vi "Dashboard Main.vi"() -> ()   [LabVIEW 2019]
uses:
  <vilib>/Utility/miscctls.llb/LVRowAndColumnTypeDef.ctl
  <vilib>/event_ctls.llb/eventvkey.ctl
  <vilib>/Rock Robotics/Network Tables/NT Read Numeric Array.vi
  <vilib>/Rock Robotics/Network Tables/NT Write Boolean.vi
  <vilib>/Rock Robotics/WPI/Dashboard/WPI_DashboardLogging Global.vi
panel:
  out "Background":bool
  in  "Camera Settings Right":T1={"Frame Rate"=30, "Compression"=30, "Size"=1, "DB Camera Config"=FALSE} {"Frame Rate" scale=1.0..30.0; "Compression" scale=100.0..-1.0; "Size" items=["640x480", "320x240", "160x120"]}
  in  "Camera Name Right":string(combo)="No Camera Selection"
  out "Camera Perf":string
  in  "Camera Settings":T1={"Frame Rate"=30, "Compression"=30, "Size"=1, "DB Camera Config"=FALSE} {"Frame Rate" scale=1.0..30.0; "Compression" scale=100.0..-1.0; "Size" items=["640x480", "320x240", "160x120"]}
  in  "TCP":refnum<k5>
  in  "Rec Mode":enum32{"Stop", "Record", "Playback"}(radio)
  out "Robot IP":string
  out "Image Message":string="Timeout in Camera Communications"
  in  "Dashboard Tab":T2(tab)
  in  "Select Auto":string(combo)="Select Autonomous ..."
  out "NT Connection":bool
  out "MotorChart R":cluster{"Numeric":dbl, "Numeric":dbl}(graph)
  out "MotorChart L":cluster{"Numeric":dbl, "Numeric":dbl}(graph)
  out "MotorSliders R":cluster{"MotorSlide1":dbl, "MotorSlide2":dbl} {"MotorSlide2" scale=-1.0..1.0 scale format="%#_2e"; "MotorSlide1" scale=-1.0..1.0 scale format="%#_2e"}
  out "MotorSliders L":cluster{"MotorSlide1":dbl, "MotorSlide2":dbl} {"MotorSlide2" scale=-1.0..1.0 scale format="%#_2e"; "MotorSlide1" scale=-1.0..1.0 scale format="%#_2e"}
  out "Gyro":dbl(knob) scale=0.0..360.0
  out "JS1 Z":dbl(slide) scale=-1.0..1.0 scale format="%#_2e"
  out "JS1 Graph":cluster{"X":dbl, "Y":dbl}[](graph)
  out "JS1 Buttons":T3
  out "JS2 Z":dbl(slide) scale=-1.0..1.0 scale format="%#_2e"
  out "JS2 Graph":cluster{"X":dbl, "Y":dbl}[](graph)
  out "JS2 Buttons":T3
  out "Mode":T4(ring)=enum."Auto Disabled"
  out "Right Camera Perf":cluster{"Bandwidth (Mbps)":dbl, "FPS":dbl}
  out "Camera Image Right":T5(plugin-control)
  in  "DB/String 9":string
  in  "DB/String 8":string
  in  "DB/String 7":string
  in  "DB/String 6":string
  in  "DB/String 5":string
  in  "DB/String 4":string
  in  "DB/String 3":string
  in  "DB/String 2":string
  in  "DB/String 1":string
  in  "DB/String 0":string
  in  "DB/Slider 0":dbl(slide) scale=0.0..5.0
  in  "DB/Slider 1":dbl(slide) scale=0.0..5.0
  in  "DB/Slider 2":dbl(slide) scale=0.0..5.0
  in  "DB/Slider 3":dbl(slide) scale=0.0..5.0
  out "DB/LED 3":bool
  out "DB/LED 2":bool
  out "DB/LED 1":bool
  out "DB/LED 0":bool
  in  "DB/Button 3":bool
  in  "DB/Button 2":bool
  in  "DB/Button 1":bool
  in  "DB/Button 0":bool caption="New Name"
  in  "OK Button":bool
  out "Danger Light":bool
  in  "Cowbell Mode":bool
  out "Hyperdrive":string
  out "Motor Mode":string
  out "Color":string
  out "Encoder 2":dbl(knob) scale=0.0..360.0
  out "Encoder 1":dbl(knob) scale=0.0..360.0
  in  "Relay":bool
  in  "Test Slider":dbl(slide) scale=0.0..100.0 scale format="%#_3g"
  in  "On/Off":bool caption="Solenoid"
  in  "Test Name":u16(ring) items=["Select the test to run..."]
  in  "Test Tree":string(tree)
  in  "Motor":cluster{"Value":dbl, "Enable":bool} {"Value" scale=-1.0..1.0 scale format="%#_3g"}
  out "Progress":T6 {"Test Progress" scale=0.0..100.0}
  in  "Rev/Fwd":cluster{"Forward":bool, "Reverse":bool}
  in  "Test Ring":u16(ring) items=["Monochrome", "Color"]
  out "Cmd Status":string
  in  "Execute Command":bool
  in  "Command Params":string[][](table)
  in  "Command Selection":i32(listbox)
  in  "CheckList":i32(listbox)
  out "Tree":string(tree)
  out "Camera Image":T5(plugin-control)
  in  "Camera Name":string(combo)="No Camera Selection"
  # "HW"
  # "HW"
  # "Joysticks"
  # "Drive Motors"
  # "Front"
  # "Right"
  # "Left"
  # "Back"
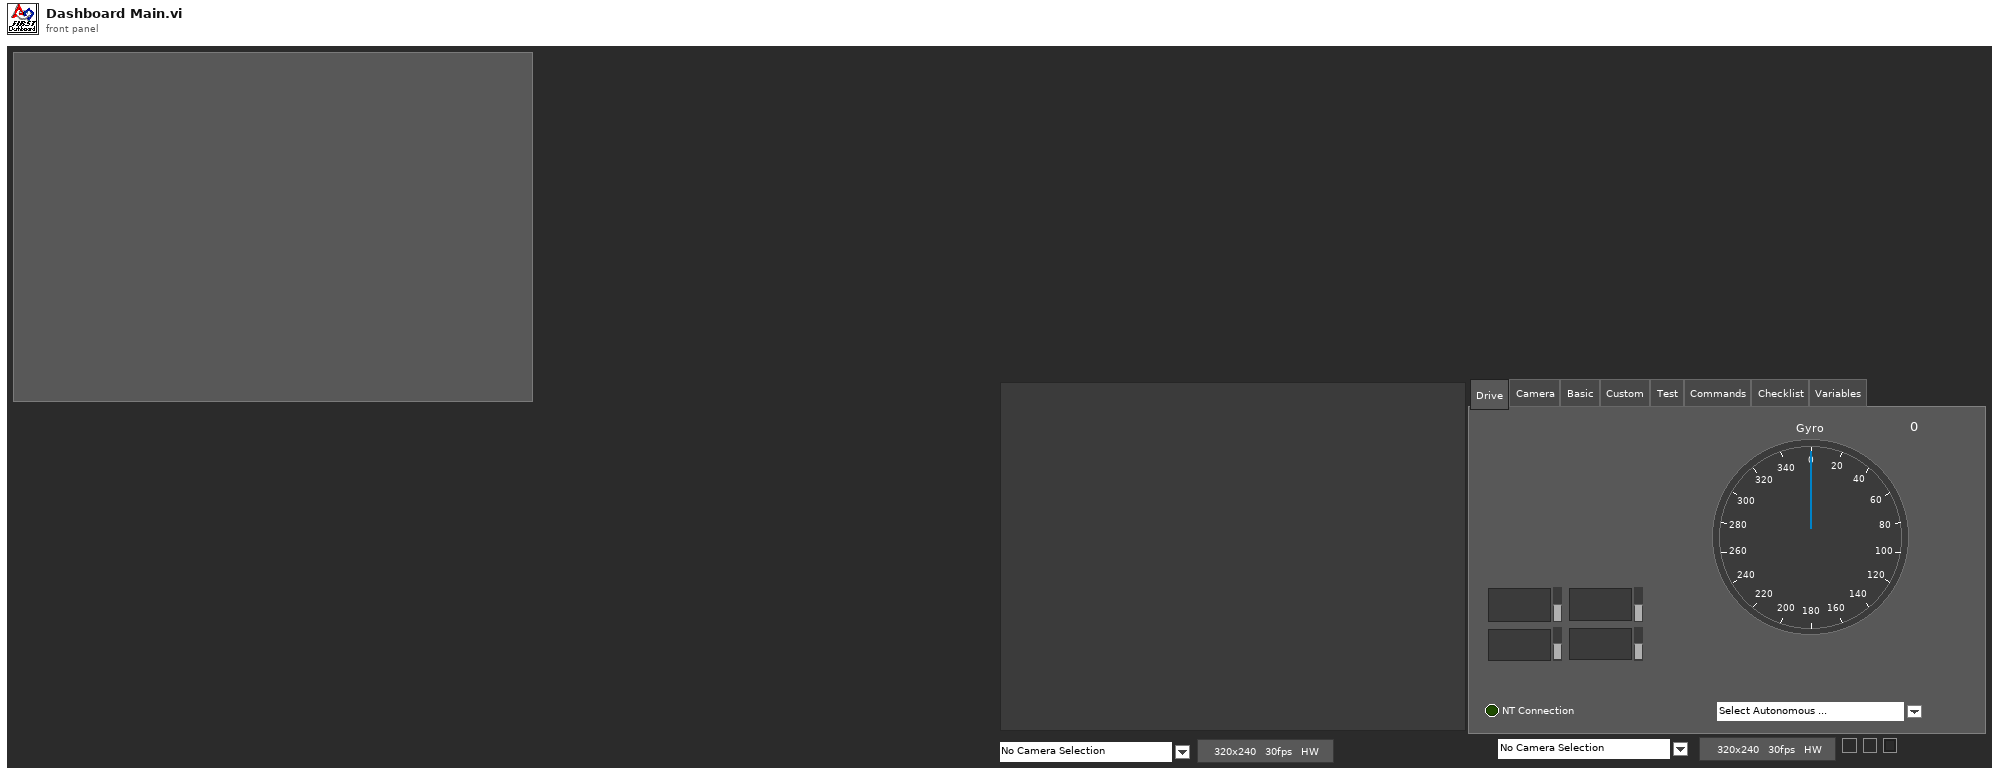
[diagram p1: front panel]
types:
  T1 = cluster{"Frame Rate":i32, "Compression":i32, "Size":u16, "DB Camera Config":bool}
  T2 = enum32{"Drive", "Camera", "Basic", "Custom", "Test", "Commands", "Checklist", "Variables"}
  T3 = cluster{bool, bool, bool, bool, bool, bool, bool, bool, bool, bool, bool, bool}
  T4 = enum8{"Tele-Op Disabled", "Tele-Op Enabled", "Auto Disabled", "Auto Enabled", "Test Disabled", "Test Enabled", "Disconnected", "No Code", "E-Stop"}
  T5 = typedef "IMAQ Image.ctl" = refnum<image>
  T6 = cluster{"Test Progress":u8, "Test Progress Text":string}
  T7 = cluster{"Save Path":path, "Interval (s)":dbl, "Keep":i32}
  T8 = typedef "Image Type" = u32
  T9 = cluster{"IDs":cluster{"RPC field ID":u16, "Unique ID":u16}, "String":string}
  T10 = cluster{"Global Rectangle":i32[], "Contours":cluster{"Contour Type":u32, "ROI Type":u32, "Points":i32[]}[]}
  T11 = cluster{"Camera Name":string, string, "Saved DB Images Info":cluster{"Save Path":path, "Interval (s)":dbl, "Keep":i32}}
  T12 = cluster{"Camera Name Right":string, string, "Saved DB Images Info":cluster{"Save Path":path, "Interval (s)":dbl, "Keep":i32}}
  T13 = cluster{"Camera Image":refnum<vi>, "Dashboard Tab":refnum<vi>, "Background":refnum<vi>, "Rec Mode":refnum<vi>, "Test Slider":refnum<vi>, "On/Off ":refnum<vi>, "Test Ring":refnum<vi>, "Rev/Fwd":refnum<vi>, "Test Name":refnum<vi>, "Motor":refnum<vi>, "Progress":refnum<vi>, "CheckList":refnum<vi>, "Tree":refnum<vi>, "Test Tree":refnum<vi>, "Command Params":refnum<vi>, "Command Selection":refnum<vi>, "Execute Command":refnum<vi>, "Cmd Status":refnum<vi>, "Camera Settings":refnum<vi>, "Camera Name":refnum<vi>, "Camera Perf":refnum<vi>, "Camera Settings Right":refnum<vi>, "Camera Name Right":refnum<vi>, "Camera Image Right":refnum<vi>}
  T14 = cluster{"Error Strings":string, "Disable Counts":cluster{u16, u16}, "Rail Faults":cluster{u16, u16, u16}, "Robot IP":string, "DB Mode":u8, "Event Info":cluster{"Name":string, "Type":u8, "Number":u16, "Replay":u8}}
  T15 = cluster{"Storage":cluster{"Disk Free":u64, "RAM Block":u32, "RAM free":u32}, "CPU Utilization":cluster{"CPU % ISR":sgl, "CPU % Time Crit":sgl, "CPU % Timed Str":sgl, "CPU % High":sgl, "CPU % Above":sgl, "CPU % Normal":sgl, "CPU % Low":sgl}, "CAN":cluster{"% Bus Utilization":sgl, "Bus Off Cnt":u32, "TX_FIFO Full Cnt":u32, "Receive Error Cnt":u8, "Transmit Error Cnt":u8}, "HID":cluster{"HID Outputs":u32, "Rumble Low":u16, "Rumble High":u16}[]}
  T16 = cluster{"Status bits":cluster{"Test Mode":bool, "Autonomous":bool, "Enabled":bool, "Code Start":bool, "Brownout":bool, "Reserved 2":bool, "Reserved 3":bool, "E-Stop":bool}, "Code Trace":cluster{"Disabled":bool, "TeleOp":bool, "Auto":bool, "Test":bool}, "Controller Type":enum16{"unknown", "cRIO", "roboRio"}, "Code?":enum16{"unknown", "noCode", "code"}, "Battery V":dbl}
  T17 = cluster{"Control Bits":cluster{"TestMode":bool, "Autonomous":bool, "Enabled":bool, "FMS Present":bool, bool, bool, bool, "E-Stop":bool}, "Team Station ":u8, "Countdown":sgl, "Joystick Values":cluster{"Axes":dbl[], "Buttons":bool[], "POVs":i16[]}[]}
  T18 = cluster{"Axes":dbl[], "Buttons":bool[], "POVs":i16[]}[]
  T19 = cluster{"Axes":dbl[], "Buttons":bool[], "POVs":i16[]}
  T20 = cluster{"Buttons[0]":bool, "Buttons[1]":bool, "Buttons[2]":bool, "Buttons[3]":bool, "Buttons[4]":bool, "Buttons[5]":bool, "Buttons[6]":bool, "Buttons[7]":bool, "Buttons[8]":bool, "Buttons[9]":bool, "Buttons[10]":bool, "Buttons[11]":bool}
  T21 = cluster{"Operation":enum16{"Update", "Clear"}, "Color Box":u32}[]
  T22 = typedef "eventvkey.ctl" = enum16{"ASCII", "Enter", "Return", "Shift", "Ctrl", "Alt", "Cmd", "Opt", "Caps", "NumLock", "Clear", "Break", "Up", "Down", "Left", "Right", "Insert", "Delete", "Home", "End", "PageUp", "PageDown", "Escape", "Help", "Pause", "ScrollLock", "F1", "F2", "F3", "F4", "F5", "F6", "F7", "F8", "F9", "F10", "F11", "F12", "F13", "F14", "F15", "F16", "F17", "F18", "F19", "F20", "F21", "F22", "F23", "F24", "Play", "VolumeUp", "VolumeDown", "Mute", "Two Byte Char"}
  T23 = cluster{"Image Size":bool, "Image Type":bool, "Pixel Value":bool, "ROI Information":bool, "Zoom Factor":bool}
  T24 = cluster{"Operation":enum16{"Update", "Clear"}, "Color Box":u32}
  T25 = typedef "LVRowAndColumnTypeDef.ctl" = cluster{"Row":i32, "Column":i32}
  T26 = cluster{"Shift":bool, "Ctrl":bool, "Alt":bool, "Cmd":bool, "Opt":bool}
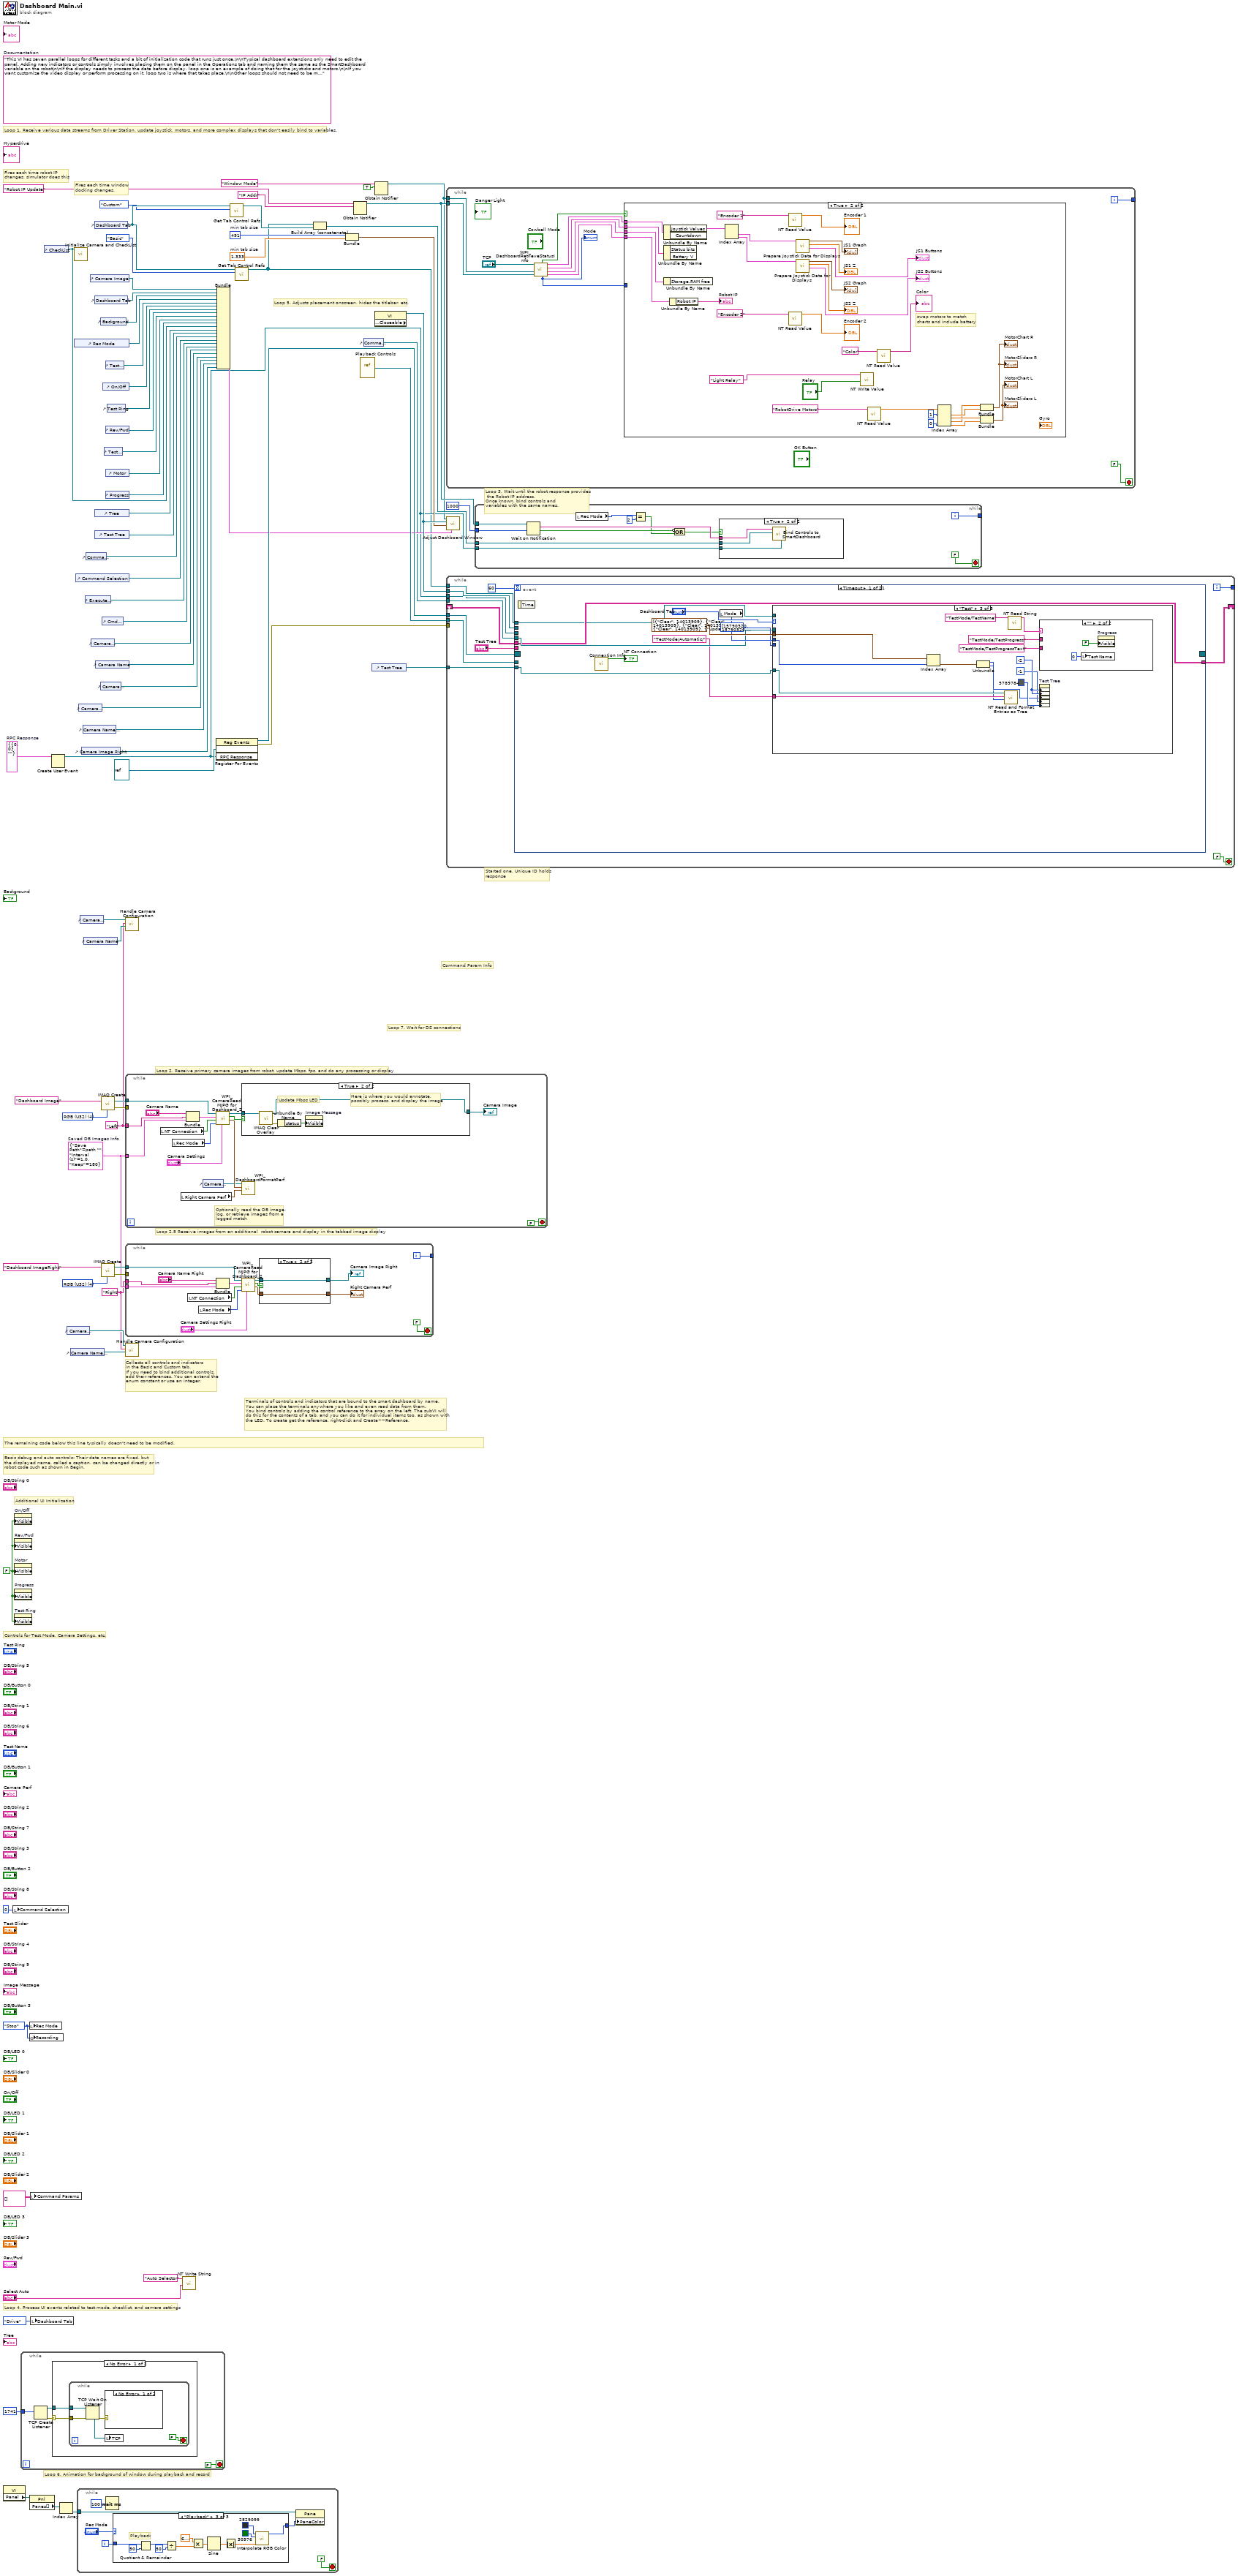
[diagram p0: block diagram]
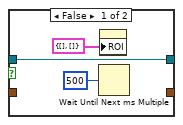
[diagram p2: hidden frame]
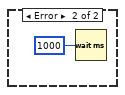
[diagram p3: hidden frame]
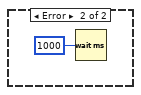
[diagram p4: hidden frame]
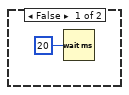
[diagram p5: hidden frame]
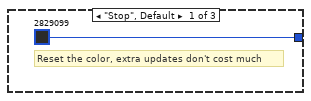
[diagram p6: hidden frame]
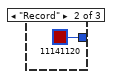
[diagram p7: hidden frame]
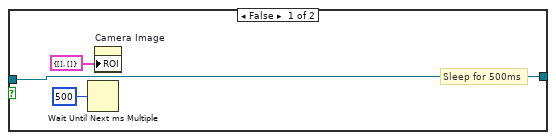
[diagram p9: hidden frame]
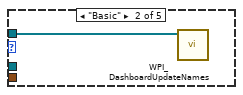
[diagram p11: hidden frame]
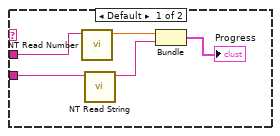
[diagram p12: hidden frame]
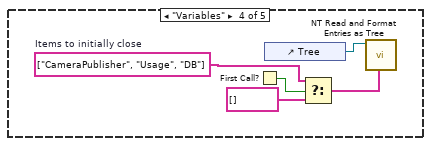
[diagram p13: hidden frame]
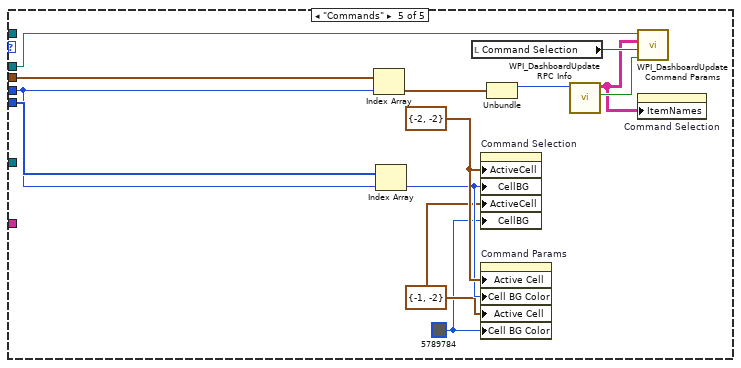
[diagram p14: hidden frame]
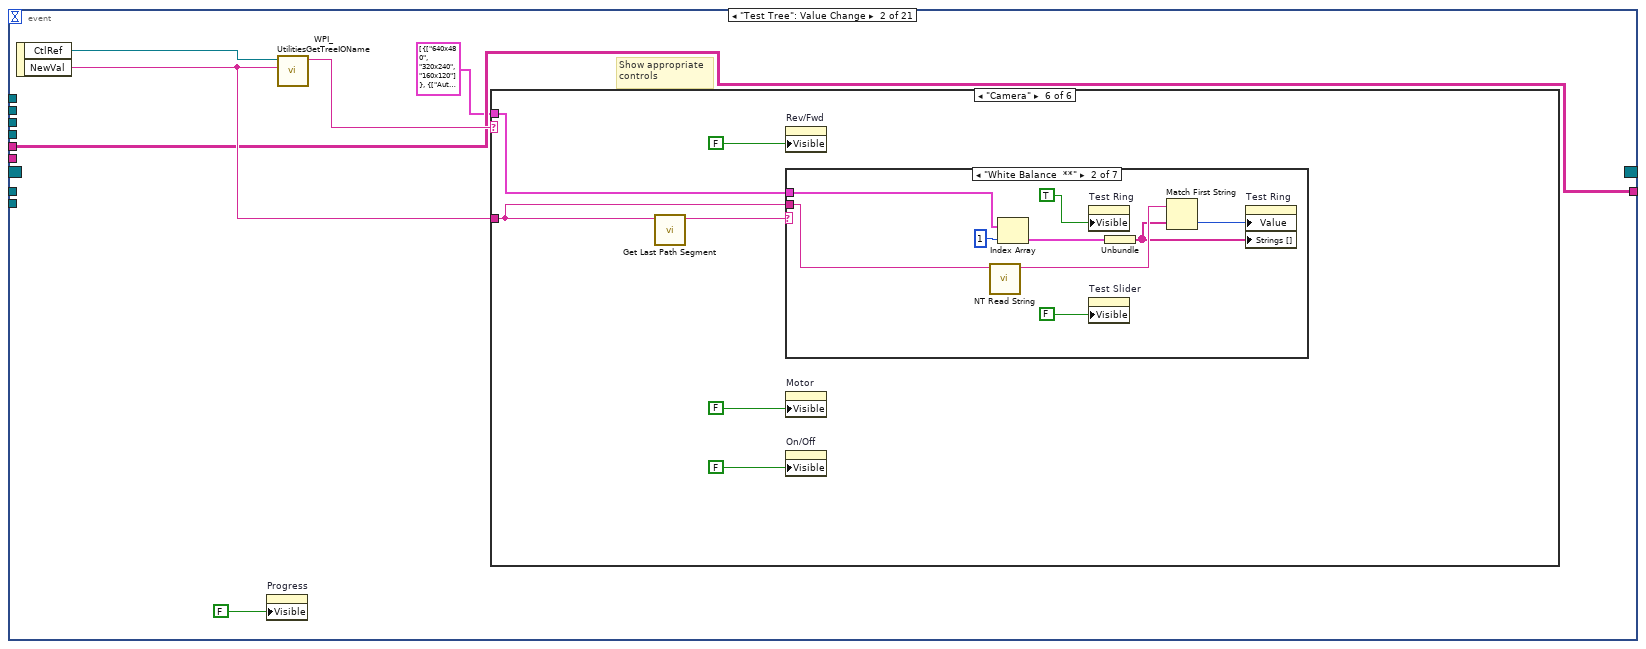
[diagram p15: hidden frame]
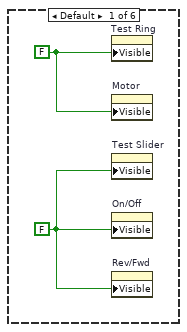
[diagram p16: hidden frame]
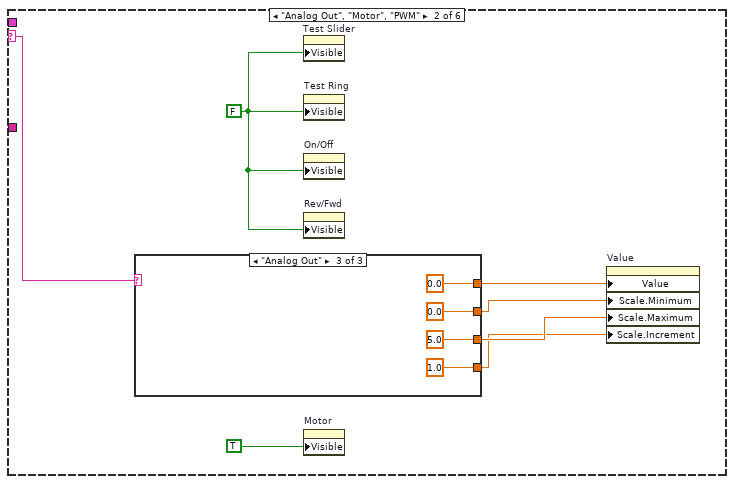
[diagram p17: hidden frame]
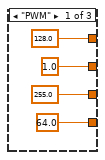
[diagram p18: hidden frame]
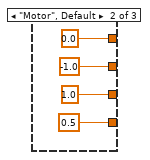
[diagram p19: hidden frame]
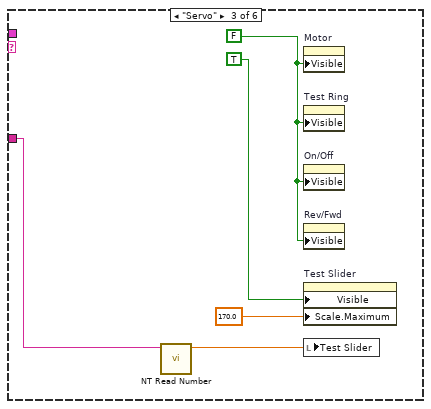
[diagram p20: hidden frame]
diagram:
  w4 = T7 {"Save Path"=path "", "Interval (s)"=1.0, "Keep"=180}  # Saved DB Images Info
  w3 = "Right"
  w2 = "Left"
  w14 = T8 4 items=["Grayscale (U8)", "Grayscale (I16)", "Grayscale (SGL)", "Complex (CSG)", "RGB (U32)", "HSL (U32)", "RGB (U64)"] ("Image Type")
  w30 = T9 {"IDs"={"RPC field ID"=0, "Unique ID"=0}, "String"=""}  # RPC Response
  w52 = 491  # min tab size
  w51 = 1.333  # min tab size
  w59 = enum32{"Stop", "Record", "Playback"}."Stop" ("Rec Mode")
  w37 = FALSE ("Visible")
  (unwired) "This VI has seven parallel loops for different tasks and a bit of initialization code that runs just once.\n\nTypical dashboard extensions only need to edit the panel. Adding new indicators or controls simply involves placing them on the panel in the Operations tab and naming them the same as the SmartDashboard variable on the robot\n\nIf the display needs to process the data before display, loop one is an example of doing that for the joysticks and motors.\n\nIf you want customize the video display or perform processing on it, loop two is where that takes place.\n\nOther loops should not need to be modified. They are pretty standard, and document the task they perform."  # Documentation
  w76 = T8 4 items=["Grayscale (U8)", "Grayscale (I16)", "Grayscale (SGL)", "Complex (CSG)", "RGB (U32)", "HSL (U32)", "RGB (U64)"] ("Image Type")
  # "Loop 2.5 Receive images from an additional  robot camera and display in the tabbed image display"
  # "Command Param Info"
  # "Started one, Unique ID holds\nresponse"
  # "Loop 7. Wait for DS connections"
  # "Basic debug and auto controls: Their data names are fixed, but\nthe displayed name, called a caption, can be changed directly or in\nrobot code such as shown in Begin."
  # "Controls for Test Mode, Camera Settings, etc."
  # "Additional UI Initialization"
  # "Loop 6. Animation for background of window during playback and record"
  # "Fires each time robot IP\nchanges, simulator does this"
  # "Fires each time window\ndocking changes."
  # "Collects all controls and indicators\nin the Basic and Custom tab.\nIf you need to bind additional controls,\nadd their references. You can extend the\nenum constant or use an integer."
  # "The remaining code below this line typically doesn't need to be modified."
  # "Loop 4. Process UI events related to test mode, checklist, and camera settings"
  # "Terminals of controls and indicators that are bound to the smart dashboard by name.\nYou can place the terminals anywhere you like and even read data from them.\nYou bind controls by adding the control reference to the array on the left. The subVI will\ndo this for the contents of a tab, and you can do it for individual items too, as shown with\nthe LED. To create get the reference, right-click and Create>>Reference."
  # "Loop 3. Wait until the robot response provides\n the Robot IP address.\nOnce known, bind controls and\nvariables with the same names."
  # "Loop 5. Adjusts placement onscreen, hides the titlebar, etc."
  # "Loop 1. Receive various data streams from Driver Station, update joystick, motors, and more complex displays that don't easily bind to variables."
  # "Loop 2. Receive primary camera images from robot, update Mbps, fps, and do any processing or display"
  n1 = property class="VI"() -> ("Panel"=w66:refnum<vi>)  [unwired: 2 in, 2 out]
  n2 = local write "Command Selection"(u16 0 ("milliseconds to wait")) -> ()
  n3 = property on="On/Off" class="Bool (strict)"("Visible"=w37) -> ()  [unwired: 2 in, 2 out]
  n4 = property on="Rev/Fwd" class="Clust (strict)"("Visible"=w37) -> ()  [unwired: 2 in, 2 out]
  n5 = property on="Motor" class="Clust (strict)"("Visible"=w37) -> ()  [unwired: 2 in, 2 out]
  n6 = property on="Progress" class="Clust (strict)"("Visible"=w37) -> ()  [unwired: 2 in, 2 out]
  n7 = property on="Test Ring" class="Ring (strict)"("Visible"=w37) -> ()  [unwired: 2 in, 2 out]
  n8 = while {
    tunnel: u16 1741 ("timeout ms (25000)") -> [w78]
    stop <- FALSE stop-if-true
    n9 = TCP Create Listener(10:w78) -> (0:w77:errorcluster, 3:w79:refnum<k5>)  [unwired: 4 in, 1 out]
    n10 = case shown="No Error" w77 {
      selector: w77 -> [w81 _]
      tunnel: w79 -> [w82 _]
      frame No Error {
        n11 = while {
          tunnel: w82 -> [w85]
          tunnel: w81 -> [w84]
          stop <- FALSE stop-if-true
          n12 = TCP Wait On Listener(8:w84, 11:w85) -> (0:w86:errorcluster, 4:w87:refnum<k5>)  [unwired: 2 in, 3 out]
          n13 = case shown="No Error" w86 {
            frame No Error {
            }
            frame Error {
              n14 = Wait (ms)(milliseconds to wait=u32 1000) -> ()  [unwired: 1 out]
            }
          }
          n15 = local write "TCP"(w87) -> ()
        }
      }
      frame Error {
        n16 = Wait (ms)(milliseconds to wait=u32 1000) -> ()  [unwired: 1 out]
      }
    }
  }
  n17 = local write "Rec Mode"(w59) -> ()
  n18 = global write "WPI_DashboardLogging Global.vi" "Recording"(w59) -> ()
  n19 = property class="Pnl"(reference=w66) -> ("Panes[]"=w67:refnum<vi>[])  [unwired: 1 in, 2 out]
  n20 = local write "Command Params"(string[][] [] ("Command Params")) -> ()
  n21 = local write "Dashboard Tab"(T2."Drive" ("Dashboard Tab")) -> ()
  n22 = control-ref of="CheckList"() -> (w48:refnum<vi>)
  n23 = Create User Event(user event datatype=w30) -> (user event=w26:refnum<user-event>)  [unwired: 1 in, 1 out]
  n24 = Index Array(array=w67) -> (element=w65:refnum<vi>)  [unwired: 1 in]
  n25 = control-ref of="Camera Settings Right"() -> (w11:refnum<vi>)
  n26 = control-ref of="Camera Name Right"() -> (w10:refnum<vi>)
  n27 = call "Initialize Camera and CheckList.vi"("ListBox in"=w48) -> ()  [unwired: 11 in]
  n28 = control-ref of="Rec Mode"() -> (w43:refnum<vi>)
  n29 = control-ref of="Command Selection"() -> (w29:refnum<vi>)
  n30 = while {
    tunnel: w65 -> [w91]
    i -> [w94]
    stop <- FALSE stop-if-true
    n31 = Wait (ms)(milliseconds to wait=u32 100) -> ()  [unwired: 1 out]
    n32 = case shown="\"Playback\"" "Rec Mode" {
      tunnel: w94 -> [_ _ w109]
      tunnel: [u32 2829099 ("Base Color") u32 11141120 ("Target Color") w98] -> w90
      frame "Stop", Default {
        # "Reset the color, extra updates don't cost much"
      }
      frame "Record" {
      }
      frame "Playback" {
        # "Playback"
        n33 = Quotient & Remainder(x=w109, y=u32 50 ("milliseconds to wait")) -> (x-y*floor(x/y)=w105:u32)  [unwired: 1 out]
        n34 = Divide(x=w105, y=u32 50 ("milliseconds to wait")) -> (x/y=w102:dbl)
        n35 = Multiply(x=6.283185307179586, y=w102) -> (x*y=w107:dbl)
        n36 = Sine(x=w107) -> (sin(x)=w106:dbl)
        n37 = Absolute Value(x=w106) -> (abs(x)=w99:dbl)
        n38 = call "Interpolate RGB Color.vi"("Proportion"=w99, "Target Color"=u32 30976, "Base Color"=u32 2829099) -> ("Result Color"=w98:u32)  [unwired: 8 in]
      }
    }
    n39 = property class="Pane"(reference=w91, "PaneColor"=w90) -> ()  [unwired: 1 in, 2 out]
  }
  n40 = control-ref of="Camera Settings Right"() -> (w9:refnum<vi>)
  n41 = control-ref of="Camera Settings"() -> (w23:refnum<vi>)
  n42 = control-ref of="Camera Image Right"() -> (w7:refnum<vi>)
  n43 = control-ref of="Camera Name Right"() -> (w8:refnum<vi>)
  n44 = control-ref of="Camera Name"() -> (w22:refnum<vi>)
  n45 = control-ref of="Execute Command"() -> (w31:refnum<vi>)
  n46 = control-ref of="Command Params"() -> (w32:refnum<vi>)
  n47 = control-ref of="Camera Image"() -> (w54:refnum<vi>)
  n48 = control-ref of="Camera Settings"() -> (w21:refnum<vi>)
  n49 = control-ref of="Dashboard Tab"() -> (w57:refnum<vi>)
  n50 = control-ref of="Dashboard Tab"() -> (w53:refnum<vi>)
  n51 = control-ref of="Tree"() -> (w47:refnum<vi>)
  n52 = control-ref of="Test Tree"() -> (w46:refnum<vi>)
  n53 = control-ref of="Camera Name"() -> (w20:refnum<vi>)
  n54 = control-ref of="Background"() -> (w1:refnum<vi>)
  n55 = control-ref of="Camera Perf"() -> (w19:refnum<vi>)
  n56 = call "IMAQ Create"("Image Name"="Dashboard Image", "Image Type"=w76) -> ("New Image"=w74:T5, "error out"=w73:errorcluster)  [unwired: 2 in, 1 out]
  n57 = call "IMAQ Create"("Image Name"="Dashboard ImageRight", "Image Type"=w14) -> ("New Image"=w13:T5, "error out"=w12:errorcluster)  [unwired: 2 in, 1 out]
  n58 = control-ref of="Cmd Status"() -> (w25:refnum<vi>)
  n59 = control-ref of="On/Off"() -> (w41:refnum<vi>)
  n60 = control-ref of="Test Name"() -> (w45:refnum<vi>)
  n61 = control-ref of="Test Slider"() -> (w42:refnum<vi>)
  n62 = control-ref of="Rev/Fwd"() -> (w39:refnum<vi>)
  n63 = control-ref of="Motor"() -> (w44:refnum<vi>)
  n64 = control-ref of="Progress"() -> (w38:refnum<vi>)
  n65 = control-ref of="Test Ring"() -> (w40:refnum<vi>)
  n66 = call "Handle Camera Configuration.vi"("CameraNameRef"=w22, "Display Name"=w2, "ClusterRef"=w23) -> ()  [unwired: 9 in]
  n67 = while {
    tunnel: w74 -> [w123]
    tunnel: w73 -> [_]
    tunnel: w4 -> [w116]
    tunnel: w2 -> [w113]
    stop <- FALSE stop-if-true
    # "Optionally read the DB image,\nlog, or retrieve images from a\nlogged match"
    n68 = local read "NT Connection"() -> (w117:bool)
    n69 = local read "Rec Mode"() -> (w120:enum32{"Stop", "Record", "Playback"})
    n70 = local read "Right Camera Perf"() -> (w111:cluster{"Bandwidth (Mbps)":dbl, "FPS":dbl})
    n71 = Bundle("Camera Name"="Camera Name", w113, "Saved DB Images Info"=w116) -> (w115:T11)  [unwired: 1 in]
    n72 = control-ref of="Camera Perf"() -> (w110:refnum<vi>)
    n73 = call <vilib>:"WPI_CameraRead MJPG for Dashboard_2.vi"("Camera Settings"="Camera Settings", "Rec Mode"=w120, "NT Connection"=w117, "Capture Info"=w115, "Image in"=w123) -> ("perf info"=w112:cluster{"Bandwidth (Mbps)":dbl, "fps":dbl}, "Active"=w121:bool, "Image\\ out"=w122:T5)  [unwired: 4 in]
    n74 = case shown="True" w121 {
      tunnel: w122 -> [w126 w129]
      tunnel: [w126 w128] -> w118
      frame False {
        # "Sleep for 500ms"
        n75 = Wait Until Next ms Multiple(millisecond multiple=u32 500) -> ()  [unwired: 1 out]
        n76 = property on="Camera Image" class="ImageControl"("ROI"=T10 {"Global Rectangle"=[], "Contours"=[]}) -> ()  [unwired: 2 in, 2 out]
      }
      frame True {
        # "Here is where you would annotate,\npossibly process, and display the image"
        # "Update Mbps LED"
        n77 = call "IMAQ Clear Overlay"("Image"=w129) -> ("error out"=w130:errorcluster, "Image Out"=w128:T5)  [unwired: 2 in, 7 out]
        n78 = Unbundle By Name(w130) -> ("status"=w131:bool)
        n79 = property on="Image Message" class="Str"("Visible"=w131) -> ()  [unwired: 2 in, 2 out]
      }
    }
    "Camera Image" <- w118
    n80 = call <vilib>:"WPI_DashboardFormatPerf.vi"("Right Camera Perf"=w111, "Performance"=w112, "String in"=w110) -> ()  [unwired: 9 in]
  }
  n81 = while {
    tunnel: w13 -> [w146]
    tunnel: w12 -> [_]
    tunnel: [w141] -> _
    tunnel: w4 -> [w137]
    tunnel: w3 -> [w134]
    i -> [w141]
    stop <- FALSE stop-if-true
    n82 = local read "NT Connection"() -> (w138:bool)
    n83 = local read "Rec Mode"() -> (w145:enum32{"Stop", "Record", "Playback"})
    n84 = Bundle("Camera Name Right"="Camera Name Right", w134, "Saved DB Images Info"=w137) -> (w136:T12)  [unwired: 1 in]
    n85 = call <vilib>:"WPI_CameraRead MJPG for Dashboard_2.vi"("Camera Settings"="Camera Settings Right", "Rec Mode"=w145, "NT Connection"=w138, "Capture Info"=w136, "Image in"=w146) -> ("perf info"=w132:cluster{"Bandwidth (Mbps)":dbl, "fps":dbl}, "Active"=w140:bool, "Image\\ out"=w143:T5)  [unwired: 4 in]
    n86 = case shown="True" w140 {
      tunnel: w143 -> [w148 w151]
      tunnel: [w148 w151] -> w139
      tunnel: [_ w150] -> w133
      tunnel: w132 -> [_ w150]
      frame False {
        n87 = Wait Until Next ms Multiple(millisecond multiple=u32 500) -> ()  [unwired: 1 out]
        n88 = property on="Camera Image Right" class="ImageControl"("ROI"=T10 {"Global Rectangle"=[], "Contours"=[]}) -> ()  [unwired: 2 in, 2 out]
      }
      frame True {
      }
    }
    "Camera Image Right" <- w139
    "Right Camera Perf" <- w133
  }
  n89 = call "Handle Camera Configuration.vi"("CameraNameRef"=w10, "Display Name"=w3, "ClusterRef"=w11) -> ()  [unwired: 9 in]
  n90 = call <vilib>:"NT Write String.vi"("String"="Select Auto", "Name"="Auto Selector") -> ()  [unwired: 9 in, 1 out]
  n91 = register-events(refnum<vi> refnum, w26) -> (reference out=w63:refnum<event-registration>, error out=w62:errorcluster)  [unwired: 2 in]
  n92 = Bundle("Camera Image"=w54, "Dashboard Tab"=w53, "Background"=w1, "Rec Mode"=w43, "Test Slider"=w42, "On/Off"=w41, "Test Ring"=w40, "Rev/Fwd"=w39, "Test Name"=w45, "Motor"=w44, "Progress"=w38, "CheckList"=w48, "Tree"=w47, "Test Tree"=w46, "Command Params"=w32, "Command Selection"=w29, "Execute Command"=w31, "Cmd Status"=w25, "Camera Settings"=w21, "Camera Name"=w20, "Camera Perf"=w19, "Camera Settings Right"=w9, "Camera Name Right"=w8, "Camera Image Right"=w7) -> (w49:T13)  [unwired: 1 in]
  n93 = call <vilib>:"Get Tab Control Refs.vi"("Page Index"=T2."Custom" ("Dashboard Tab"), "TabControl in"=w57) -> ("ControlsOnPage"=w56:refnum<vi>[])  [unwired: 9 in]
  n94 = call <vilib>:"Get Tab Control Refs.vi"("Page Index"=T2."Basic" ("Dashboard Tab"), "TabControl in"=w57) -> ("ControlsOnPage"=w18:refnum<vi>[])  [unwired: 9 in]
  n95 = Build Array (concatenate)(w18, w56) -> (w55:refnum<vi>[])
  n96 = Bundle("min tab size"=w52, "min tab size"=w51) -> (w50:cluster{"min tab size":i32, "min tab size":dbl})  [unwired: 1 in]
  n97 = Obtain Notifier(name (unnamed)="Robot IP Update", notification data type="IP Addr" ("name (unnamed)")) -> (notifier out=w36:refnum<notifier>)  [unwired: 2 in, 2 out]
  n98 = vi-ref "Playback Controls.vi"() -> (w64:refnum<vi>)
  n99 = control-ref of="Command Params"() -> (w24:refnum<vi>)
  n100 = control-ref of="Test Tree"() -> (w68:refnum<vi>)
  n101 = property class="VI" props=["Front Panel.Closeable"]() -> (reference out=w58:refnum<vi>)  [unwired: 2 in, 2 out]
  n102 = Obtain Notifier(name (unnamed)="Window Mode", notification data type=TRUE) -> (notifier out=w35:refnum<notifier>)  [unwired: 2 in, 2 out]
  n103 = while {
    tunnel: [w161] -> _
    tunnel: w36 -> [w155]
    tunnel: w35 -> [w152]
    i -> [w161]
    stop <- FALSE stop-if-true
    n104 = call <vilib>:"WPI_DashboardRetrieveStatusInfo.vi"("Binding Refnum"=w155, "Window Mode Notifier"=w152, "TCP Cnx"="TCP") -> ("Power and Errors"=w156:T14, "Robot Metrics"=w159:T15, "Status Info"=w160:T16, "Control Info"=w157:T17, "Robot Mode"=w154:T4, "Process?"=w158:bool)  [unwired: 3 in]
    "Mode" <- w154
    n105 = case shown="True" w158 {
      tunnel: w160 -> [_ w195]
      tunnel: w159 -> [_ w194]
      tunnel: w157 -> [_ w193]
      tunnel: w156 -> [_ w192]
      tunnel: w154 -> [_ _]
      frame False {
        n106 = Wait (ms)(milliseconds to wait=u32 20) -> ()  [unwired: 1 out]
      }
      frame True {
        # "swap motors to match\ncharts and include battery"
        n107 = Unbundle By Name(w193) -> ("Joystick Values"=w183:T18)  [unwired: 1 out]
        n108 = Unbundle By Name(w195) -> ()  [unwired: 2 out]
        n109 = Unbundle By Name(w194) -> ()  [unwired: 1 out]
        n110 = Unbundle By Name(w192) -> ("Robot IP"=→"Robot IP":string)
        n111 = Index Array(array=w183) -> (element #1=w182:T19, element #2=w178:T19)  [unwired: 2 in]
        n112 = call-poly <vilib>:"NT Read Value.vi"("Name"="Encoder 1") -> ("Numeric"=→"Encoder 1":dbl)  [unwired: 9 in, 1 out]
        n113 = call-poly <vilib>:"NT Read Value.vi"("Name"="Encoder 2") -> ("Numeric"=→"Encoder 2":dbl)  [unwired: 9 in, 1 out]
        n114 = call "Prepare Joystick Data for Displays.vi"("Joystick Values"=w182) -> ("Buttons"=→"JS1 Buttons":T20, "Z Axis"=→"JS1 Z":dbl, "Cartesian Data"=→"JS1 Graph":cluster{"X axis":dbl, "X axis":dbl}[])  [unwired: 8 in]
        n115 = call "Prepare Joystick Data for Displays.vi"("Joystick Values"=w178) -> ("Buttons"=→"JS2 Buttons":T20, "Z Axis"=→"JS2 Z":dbl, "Cartesian Data"=→"JS2 Graph":cluster{"X axis":dbl, "X axis":dbl}[])  [unwired: 8 in]
        n116 = call-poly <vilib>:"NT Write Value.vi"("Boolean"="Relay", "Name"="Light Relay") -> ()  [unwired: 9 in, 1 out]
        n117 = call-poly <vilib>:"NT Read Value.vi"("Name"="RobotDrive Motors") -> ("Numeric Array"=w173:dbl[])  [unwired: 9 in, 1 out]
        n118 = call-poly <vilib>:"NT Read Value.vi"("Name"="Color") -> ("String"=→"Color":string)  [unwired: 9 in, 1 out]
        n119 = Index Array(array=w173, index #1=1, index #4=0) -> (element #1=w187:dbl, element #2=w188:dbl, element #3=w186:dbl, element #4=w191:dbl)  [unwired: 2 in]
        n120 = Bundle("Numeric"=w186, "Numeric"=w187) -> (→"MotorChart R" →"MotorSliders R":cluster{"Numeric":dbl, "Numeric":dbl})  [unwired: 1 in]
        n121 = Bundle("Numeric"=w188, "Numeric"=w191) -> (→"MotorChart L" →"MotorSliders L":cluster{"Numeric":dbl, "Numeric":dbl})  [unwired: 1 in]
      }
    }
  }
  n122 = call "Adjust Dashboard Window.vi"("Sizing Refnums"=w49, "Size Constraints"=w50, "VI"=w58, "WIn Mode"=w35) -> ()  [unwired: 8 in]
  n123 = while {
    tunnel: [w205] -> _
    tunnel: w68 -> [w204]
    tunnel: w64 -> [w203]
    tunnel: w63 -> [w202]
    tunnel: w62 -> [_]
    tunnel: w58 -> [w201]
    tunnel: w26 -> [w200]
    tunnel: w24 -> [w199]
    shift-right: [w198] -> _
    shift-left: _ -> [w197]
    tunnel: w18 -> [w196]
    i -> [w205]
    stop <- FALSE stop-if-true
    n124 = event shown="[0] Timeout" {
      selector: w202 -> [_ _ _ _ _ _ _ _ _ _ _ _ _ _ _ _ _ _ _ _ _]
      dyn-events: [_ _ _ _ _ _ _ _ _ _ _ _ _ _ _ _ w465 _ _ _ _] -> _
      timeout: u32 60 ("milliseconds to wait") -> [_ _ _ _ _ _ _ _ _ _ _ _ _ _ _ _ _ _ _ _ _]
      tunnel: w204 -> [w217 _ _ _ _ _ _ _ _ _ _ _ _ _ _ _ _ _ _ _ _]
      tunnel: "Test Tree" -> [_ _ _ _ _ _ _ _ _ _ _ w432 w440 w442 w446 w454 _ _ _ _ _]
      tunnel: w203 -> [_ _ _ _ _ _ _ _ _ _ _ _ _ _ _ _ w467 _ w485 _ _]
      tunnel: w201 -> [_ _ _ _ _ _ _ _ _ _ _ _ _ _ _ _ w463 _ _ _ _]
      tunnel: w200 -> [_ _ _ _ _ _ _ _ _ _ _ _ _ _ _ _ w461 _ _ _ _]
      tunnel: w199 -> [w212 _ _ _ _ _ w383 _ _ _ _ _ _ _ _ _ _ _ _ _ _]
      tunnel: [w211 w260 w362 w367 w376 w380 w381 w390 w400 w407 w419 w431 w438 w441 w445 w453 w460 w480 w482 w486 w499] -> w198
      tunnel: w197 -> [w211 w260 w362 w367 w376 w380 w381 _ _ w407 w419 w431 w438 w441 w445 w453 w460 w480 w482 w486 w499]
      tunnel: w196 -> [w209 _ _ _ _ _ _ _ _ _ _ _ _ _ _ _ _ _ _ _ _]
      event Timeout {
        n125 = event-data() -> ()  [unwired: 1 in, 1 out]
        n126 = call <vilib>:"Connextion Info.vi"() -> ("Connected"=→"NT Connection":bool)  [unwired: 10 in, 1 out]
        n127 = local read "Mode"() -> (w214:T4)
        n128 = case shown="\"Test\"" "Dashboard Tab" {
          tunnel: w217 -> [_ _ w233 _ _]
          tunnel: "TestMode/Automatic/" ("Name Pattern") -> [_ _ w232 _ _]
          tunnel: T21 [{"Operation"=enum."Clear", "Color Box"=14013909}, {"Operation"=enum."Clear", "Color Box"=14013909}, {"Operation"=enum."Clear", "Color Box"=14013909}, {"Operation"=enum."Clear", "Color Box"=14013909}, {"Operation"=enum."Update", "Color Box"=14013909}, {"Operation"=enum."Update", "Color Box"=16777215}, {"Operation"=enum."Clear", "Color Box"=14013909}, {"Operation"=enum."Clear", "Color Box"=14013909}, {"Operation"=enum."Clear", "Color Box"=14013909}] -> [_ _ w225 _ w253]
          tunnel: w214 -> [_ _ w224 _ w252]
          tunnel: u32[] [15790320, 15790320, 15790320, 15790320, 16777215, 16777215, 15790320, 15790320, 15790320] -> [_ _ _ _ w258]
          tunnel: w212 -> [_ _ _ _ w246]
          tunnel: w209 -> [_ w219 _ _ _]
          frame "Custom", Default {
          }
          frame "Basic" {
            n129 = call <vilib>:"WPI_DashboardUpdateNames.vi"("Controls on Tab"=w219) -> ()  [unwired: 11 in]
          }
          frame "Test" {
            w231 = -2 ("Active Item:Row Number")
            n130 = Index Array(array=w225, index=w224) -> (element=w226:T24)
            n131 = Unbundle(w226) -> ("Operation"=w227:enum16{"Update", "Clear"}, "Color Box"=w228:u32)
            n132 = call <vilib>:"NT Read and Format Entries as Tree.vi"("Operation"=w227, "Name Pattern"=w232, "Tree Refnum"=w233) -> ()  [unwired: 7 in, 2 out]
            n133 = call <vilib>:"NT Read String.vi"("Name"="TestMode/TestName") -> ("String"=w222:string)  [unwired: 9 in, 1 out]
            n134 = case shown="\"\"" w222 {
              tunnel: "TestMode/TestProgress" ("Name") -> [w235 _]
              tunnel: "TestMode/TestProgressText" ("Name") -> [w234 _]
              frame Default {
                n135 = call <vilib>:"NT Read Number.vi"("Name"=w235) -> ("Numeric"=w236:dbl)  [unwired: 9 in, 1 out]
                n136 = call <vilib>:"NT Read String.vi"("Name"=w234) -> ("String"=w237:string)  [unwired: 9 in, 1 out]
                n137 = Bundle("Numeric"=w236, "String"=w237) -> (→"Progress":cluster{"Numeric":dbl, "String":string})  [unwired: 1 in]
              }
              frame "" {
                n138 = local write "Test Name"(u16 0) -> ()
                n139 = property on="Progress" class="Clust (strict)"("Visible"=FALSE) -> ()  [unwired: 2 in, 2 out]
              }
            }
            n140 = property on="Test Tree" class="Tree (strict)"("Active Item Row Number"=w231, "ActiveColNum"=w231, "CellBG"=w228, "Active Item Row Number"=-1 ("Active Item:Row Number"), "CellBG"=u32 5789784 ("Color Box")) -> ()  [unwired: 2 in, 2 out]
          }
          frame "Variables" {
            w243 = string[] ["CameraPublisher", "Usage", "DB"]  # Items to initially close
            n141 = First Call?() -> (First Call?: T/F=w244:bool)
            n142 = control-ref of="Tree"() -> (w245:refnum<vi>)
            n143 = Select(t=w243, s=w244, f=string[] []) -> (s? t:f=w241:string[])
            n144 = call <vilib>:"NT Read and Format Entries as Tree.vi"("Tags to  Close"=w241, "Tree Refnum"=w245) -> ()  [unwired: 8 in, 2 out]
          }
          frame "Commands" {
            w254 = u32 5789784 ("Color Box")
            w255 = T25 {"Row"=-1, "Column"=-2} ("Active Cell:Active Cell")
            w257 = T25 {"Row"=-2, "Column"=-2} ("Active Cell:Active Cell")
            n145 = Index Array(array=w253, index=w252) -> (element=w251:T24)
            n146 = Index Array(array=w258, index=w252) -> (element=w256:u32)
            n147 = local read "Command Selection"() -> (w249:i32)
            n148 = property on="Command Selection" class="MCListbox (strict)"("ActiveCell"=w257, "CellBG"=w256, "ActiveCell"=w255, "CellBG"=w254) -> ()  [unwired: 2 in, 2 out]
            n149 = property on="Command Params" class="Tbl (strict)"("Active Cell"=w257, "Cell BG Color"=w256, "Active Cell"=w255, "Cell BG Color"=w254) -> ()  [unwired: 2 in, 2 out]
            n150 = Unbundle(w251) -> ("Operation"=w250:enum16{"Update", "Clear"})  [unwired: 1 out]
            n151 = call <vilib>:"WPI_DashboardUpdate RPC Info.vi"("Operation"=w250) -> ("update"=w248:bool, "commands"=w247:string[][])  [unwired: 9 in]
            n152 = call <vilib>:"WPI_DashboardUpdate Command Params.vi"("Update"=w248, "NewVal"=w249, "Commands"=w247, "Param Tbl"=w246) -> ()  [unwired: 7 in, 1 out]
            n153 = property on="Command Selection" class="MCListbox (strict)"("ItemNames"=w247) -> ()  [unwired: 2 in, 2 out]
          }
        }
      }
      event "Test Tree": Value Change {
        # "Show appropriate\ncontrols"
        n154 = event-data() -> ("CtlRef"=w263:refnum<vi>, "NewVal"=w261:string)  [unwired: 1 in]
        n155 = property on="Progress" class="Clust (strict)"("Visible"=FALSE) -> ()  [unwired: 2 in, 2 out]
        n156 = call <vilib>:"WPI_UtilitiesGetTreeIOName.vi"("NewVal"=w261, "TreeControl in"=w263) -> ("I/O Name"=w264:string)  [unwired: 9 in]
        n157 = case shown="\"Camera\"" w264 {
          selector: w264 -> [_ w271 _ w293 w302 _]
          tunnel: w261 -> [_ _ w290 w292 _ w309]
          tunnel: cluster{string[]}[] [{["640x480", "320x240", "160x120"]}, {["Auto", "Fixed indoor", "Fixed outdoor 1", "Fixed outdoor 2", "Fixed fluorescent 1", "Fixed fluorescent 2", "Hold current"]}, {["Auto", "Flicker-free 50 Hz", "Flicker-free 60 Hz", "Hold current"]}, {["None", "Prioritize frame rate", "Prioritize image quality"]}, {["Monochrome", "Color"]}] -> [_ _ _ _ _ w308]
          frame Default {
            w266 = FALSE ("Visible")
            w265 = FALSE ("Visible")
            n158 = property on="Test Ring" class="Ring (strict)"("Visible"=w265) -> ()  [unwired: 2 in, 2 out]
            n159 = property on="Motor" class="Clust (strict)"("Visible"=w265) -> ()  [unwired: 2 in, 2 out]
            n160 = property on="Test Slider" class="Slide (strict)"("Visible"=w266) -> ()  [unwired: 2 in, 2 out]
            n161 = property on="On/Off" class="Bool (strict)"("Visible"=w266) -> ()  [unwired: 2 in, 2 out]
            n162 = property on="Rev/Fwd" class="Clust (strict)"("Visible"=w266) -> ()  [unwired: 2 in, 2 out]
          }
          frame "Analog Out", "Motor", "PWM" {
            w272 = FALSE ("Visible")
            n163 = case shown="\"Analog Out\"" w271 {
              tunnel: [1.0 ("Value") -1.0 ("Value") 0.0 ("Value")] -> w270
              tunnel: [255.0 ("Value") 1.0 ("Value") 5.0 ("Value")] -> w269
              tunnel: [128.0 ("Value") 0.0 ("Value") 0.0 ("Value")] -> w268
              tunnel: [64.0 ("Value") 0.5 ("Value") 1.0 ("Value")] -> w267
              frame "PWM" {
              }
              frame "Motor", Default {
              }
              frame "Analog Out" {
              }
            }
            n164 = property on="Test Slider" class="Slide (strict)"("Visible"=w272) -> ()  [unwired: 2 in, 2 out]
            n165 = property on="Test Ring" class="Ring (strict)"("Visible"=w272) -> ()  [unwired: 2 in, 2 out]
            n166 = property on="On/Off" class="Bool (strict)"("Visible"=w272) -> ()  [unwired: 2 in, 2 out]
            n167 = property on="Rev/Fwd" class="Clust (strict)"("Visible"=w272) -> ()  [unwired: 2 in, 2 out]
            n168 = property on="Motor" class="Clust (strict)"("Visible"=TRUE) -> ()  [unwired: 2 in, 2 out]
            n169 = property on="Value" class="Slide (strict)"("Value"=w268, "Scale.Minimum"=w270, "Scale.Maximum"=w269, "Scale.Increment"=w267) -> ()  [unwired: 2 in, 2 out]
          }
          frame "Servo" {
            w288 = FALSE ("Visible")
            n170 = call <vilib>:"NT Read Number.vi"("Name"=w290) -> ("Numeric"=w289:dbl)  [unwired: 9 in, 1 out]
            n171 = property on="Motor" class="Clust (strict)"("Visible"=w288) -> ()  [unwired: 2 in, 2 out]
            n172 = property on="Test Ring" class="Ring (strict)"("Visible"=w288) -> ()  [unwired: 2 in, 2 out]
            n173 = property on="On/Off" class="Bool (strict)"("Visible"=w288) -> ()  [unwired: 2 in, 2 out]
            n174 = property on="Rev/Fwd" class="Clust (strict)"("Visible"=w288) -> ()  [unwired: 2 in, 2 out]
            n175 = property on="Test Slider" class="Slide (strict)"("Visible"=TRUE, "Scale.Maximum"=170.0 ("Scale.Range:Maximum")) -> ()  [unwired: 2 in, 2 out]
            n176 = local write "Test Slider"(w289) -> ()
          }
          frame "Relay", "Solenoid" {
            w291 = FALSE ("Visible")
            n177 = property on="Motor" class="Clust (strict)"("Visible"=w291) -> ()  [unwired: 2 in, 2 out]
            n178 = property on="Test Slider" class="Slide (strict)"("Visible"=w291) -> ()  [unwired: 2 in, 2 out]
            n179 = property on="Test Ring" class="Ring (strict)"("Visible"=w291) -> ()  [unwired: 2 in, 2 out]
            n180 = Search and Replace String(input string=w292, search string="/Value  **", replace string="/Direction") -> (result string=w298:string)  [unwired: 5 in, 3 out]
            n181 = call <vilib>:"NT Read String.vi"("Name"=w298) -> ("String"=w296:string)  [unwired: 9 in, 1 out]
            n182 = Equal?(x="Both directions", y=w296) -> (x = y?=w294:bool)
            n183 = property on="Rev/Fwd" class="Clust (strict)"("Visible"=w294) -> ()  [unwired: 2 in, 2 out]
            n184 = Not(x=w294) -> (.not. x?=w295:bool)
            n185 = property on="On/Off" class="Bool (strict)"("Visible"=w295, "Caption.Text"=w293) -> ()  [unwired: 2 in, 2 out]
          }
          frame "Compressor", "Digital Out" {
            w301 = FALSE ("Visible")
            # "Get direction and finish"
            n186 = property on="Test Ring" class="Ring (strict)"("Visible"=w301) -> ()  [unwired: 2 in, 2 out]
            n187 = property on="Motor" class="Clust (strict)"("Visible"=w301) -> ()  [unwired: 2 in, 2 out]
            n188 = property on="Test Slider" class="Slide (strict)"("Visible"=w301) -> ()  [unwired: 2 in, 2 out]
            n189 = property on="Rev/Fwd" class="Clust (strict)"("Visible"=FALSE) -> ()  [unwired: 2 in, 2 out]
            n190 = property on="On/Off" class="Bool (strict)"("Visible"=TRUE, "Caption.Text"=w302) -> ()  [unwired: 2 in, 2 out]
          }
          frame "Camera" {
            n191 = call <vilib>:"Get Last Path Segment.vi"("String in"=w309) -> ("String out"=w310:string)  [unwired: 10 in]
            n192 = property on="Rev/Fwd" class="Clust (strict)"("Visible"=FALSE) -> ()  [unwired: 2 in, 2 out]
            n193 = case shown="\"White Balance  **\"" w310 {
              tunnel: w309 -> [w316 w325 w334 w343 w352 _ w358]
              tunnel: w308 -> [w314 w322 w331 w340 w349 _ _]
              frame "Size  **" {
                n194 = Index Array(array=w314) -> (element=w313:cluster{string[]})  [unwired: 1 in]
                n195 = call <vilib>:"NT Read String.vi"("Name"=w316) -> ("String"=w315:string)  [unwired: 9 in, 1 out]
                n196 = property on="Test Ring" class="Ring (strict)"("Visible"=TRUE) -> ()  [unwired: 2 in, 2 out]
                n197 = property on="Test Slider" class="Slide (strict)"("Visible"=FALSE) -> ()  [unwired: 2 in, 2 out]
                n198 = Unbundle(w313) -> (w311:string[])
                n199 = Match First String(2:w311, 3:w315) -> (0:w312:i32)  [unwired: 1 out]
                n200 = property on="Test Ring" class="Ring (strict)"("Value"=w312, "Strings []"=w311) -> ()  [unwired: 2 in, 2 out]
              }
              frame "White Balance  **" {
                n201 = call <vilib>:"NT Read String.vi"("Name"=w325) -> ("String"=w324:string)  [unwired: 9 in, 1 out]
                n202 = Index Array(array=w322, index=1) -> (element=w323:cluster{string[]})
                n203 = property on="Test Ring" class="Ring (strict)"("Visible"=TRUE) -> ()  [unwired: 2 in, 2 out]
                n204 = property on="Test Slider" class="Slide (strict)"("Visible"=FALSE) -> ()  [unwired: 2 in, 2 out]
                n205 = Unbundle(w323) -> (w320:string[])
                n206 = Match First String(2:w320, 3:w324) -> (0:w319:i32)  [unwired: 1 out]
                n207 = property on="Test Ring" class="Ring (strict)"("Value"=w319, "Strings []"=w320) -> ()  [unwired: 2 in, 2 out]
              }
              frame "Exposure  **" {
                n208 = call <vilib>:"NT Read String.vi"("Name"=w334) -> ("String"=w333:string)  [unwired: 9 in, 1 out]
                n209 = Index Array(array=w331, index=2) -> (element=w332:cluster{string[]})
                n210 = property on="Test Ring" class="Ring (strict)"("Visible"=TRUE) -> ()  [unwired: 2 in, 2 out]
                n211 = property on="Test Slider" class="Slide (strict)"("Visible"=FALSE) -> ()  [unwired: 2 in, 2 out]
                n212 = Unbundle(w332) -> (w328:string[])
                n213 = Match First String(2:w328, 3:w333) -> (0:w329:i32)  [unwired: 1 out]
                n214 = property on="Test Ring" class="Ring (strict)"("Value"=w329, "Strings []"=w328) -> ()  [unwired: 2 in, 2 out]
              }
              frame "Exposure Priority  **" {
                n215 = call <vilib>:"NT Read String.vi"("Name"=w343) -> ("String"=w342:string)  [unwired: 9 in, 1 out]
                n216 = Index Array(array=w340, index=3) -> (element=w341:cluster{string[]})
                n217 = property on="Test Ring" class="Ring (strict)"("Visible"=TRUE) -> ()  [unwired: 2 in, 2 out]
                n218 = property on="Test Slider" class="Slide (strict)"("Visible"=FALSE) -> ()  [unwired: 2 in, 2 out]
                n219 = Unbundle(w341) -> (w337:string[])
                n220 = Match First String(2:w337, 3:w342) -> (0:w338:i32)  [unwired: 1 out]
                n221 = property on="Test Ring" class="Ring (strict)"("Value"=w338, "Strings []"=w337) -> ()  [unwired: 2 in, 2 out]
              }
              frame "Color Enable  **" {
                n222 = call <vilib>:"NT Read String.vi"("Name"=w352) -> ("String"=w351:string)  [unwired: 9 in, 1 out]
                n223 = Index Array(array=w349, index=4) -> (element=w350:cluster{string[]})
                n224 = property on="Test Ring" class="Ring (strict)"("Visible"=TRUE) -> ()  [unwired: 2 in, 2 out]
                n225 = property on="Test Slider" class="Slide (strict)"("Visible"=FALSE) -> ()  [unwired: 2 in, 2 out]
                n226 = Unbundle(w350) -> (w346:string[])
                n227 = Match First String(2:w346, 3:w351) -> (0:w347:i32)  [unwired: 1 out]
                n228 = property on="Test Ring" class="Ring (strict)"("Value"=w347, "Strings []"=w346) -> ()  [unwired: 2 in, 2 out]
              }
              frame Default {
                n229 = property on="Test Slider" class="Slide (strict)"("Visible"=FALSE) -> ()  [unwired: 2 in, 2 out]
                n230 = property on="Test Ring" class="Ring (strict)"("Visible"=FALSE) -> ()  [unwired: 2 in, 2 out]
              }
              frame "Brightness  **", "Color Level  **", "Compression  **", "FPS  **", "Sharpness  **" {
                n231 = call <vilib>:"NT Read Number.vi"("Name"=w358) -> ("Numeric"=w357:dbl)  [unwired: 9 in, 1 out]
                n232 = property on="Test Ring" class="Ring (strict)"("Visible"=FALSE) -> ()  [unwired: 2 in, 2 out]
                n233 = property on="Test Slider" class="Slide (strict)"("Visible"=TRUE, "Scale.Maximum"=100.0 ("Scale.Range:Maximum")) -> ()  [unwired: 2 in, 2 out]
                n234 = local write "Test Slider"(w357) -> ()
              }
            }
            n235 = property on="Motor" class="Clust (strict)"("Visible"=FALSE) -> ()  [unwired: 2 in, 2 out]
            n236 = property on="On/Off" class="Bool (strict)"("Visible"=FALSE) -> ()  [unwired: 2 in, 2 out]
          }
        }
      }
      event "Test Name": Mouse Enter {
        # "Populate the ring with the list of tests"
        n237 = event-data() -> ()  [unwired: 1 in, 1 out]
        n238 = call <vilib>:"NT Read String Array.vi"("Name"="TestMode/TestList") -> ("String Array"=w366:string[])  [unwired: 9 in, 1 out]
        n239 = Build Array (concatenate)("Select the test to run...", w366) -> (w365:string[])
        n240 = property on="Test Name" class="Ring (strict)"("Strings []"=w365) -> ()  [unwired: 2 in, 2 out]
      }
      event "Test Name": Value Change {
        w368 = FALSE ("Visible")
        # "Tell the robot the test name to run"
        n241 = event-data() -> ("NewVal"=w372:u16)  [unwired: 1 in]
        n242 = property on="Test Name" class="Ring (strict)"() -> ("Strings []"=w373:string[])  [unwired: 2 in, 2 out]
        n243 = property on="Progress" class="Clust (strict)"("Visible"=TRUE) -> ()  [unwired: 2 in, 2 out]
        n244 = local write "Progress"(T6 {"Test Progress"=0, "Test Progress Text"=""} ("Progress")) -> ()
        n245 = property on="Test Ring" class="Ring (strict)"("Visible"=w368) -> ()  [unwired: 2 in, 2 out]
        n246 = property on="Motor" class="Clust (strict)"("Visible"=w368) -> ()  [unwired: 2 in, 2 out]
        n247 = property on="Test Slider" class="Slide (strict)"("Visible"=w368) -> ()  [unwired: 2 in, 2 out]
        n248 = property on="On/Off" class="Bool (strict)"("Visible"=w368) -> ()  [unwired: 2 in, 2 out]
        n249 = property on="Rev/Fwd" class="Clust (strict)"("Visible"=w368) -> ()  [unwired: 2 in, 2 out]
        n250 = Index Array(array=w373, index=w372) -> (element=w371:string)
        n251 = call <vilib>:"NT Write String.vi"("String"=w371, "Name"="TestMode/TestName") -> ()  [unwired: 9 in, 1 out]
      }
      event "Select Auto": Mouse Enter {
        # "Populate the combo box with the list of autonomous options"
        n252 = event-data() -> ()  [unwired: 1 in, 1 out]
        n253 = call <vilib>:"NT Read String Array.vi"("Name"="Auto List") -> ("String Array"=w375:string[])  [unwired: 9 in, 1 out]
        n254 = property on="Select Auto" class="CmbBox"("Strings[]"=w375) -> ()  [unwired: 2 in, 2 out]
      }
      event "Select Auto": Value Change {
        # "User modified the Auto Selection. Write to NT variable so robot knows."
        n255 = event-data() -> ("NewVal"=w378:string)  [unwired: 1 in]
        n256 = call <vilib>:"NT Write String.vi"("String"=w378, "Name"="Auto Selector") -> ()  [unwired: 9 in, 1 out]
      }
      event "Command Selection": Value Change {
        # "Get the params and show in table"
        n257 = event-data() -> ("NewVal"=w384:i32)  [unwired: 1 in]
        n258 = property on="Command Selection" class="MCListbox (strict)"() -> ("ItemNames"=w382:string[][])  [unwired: 2 in, 2 out]
        n259 = call <vilib>:"WPI_DashboardUpdate Command Params.vi"("NewVal"=w384, "Commands"=w382, "Param Tbl"=w383) -> ()  [unwired: 8 in, 1 out]
      }
      event "Execute Command": Value Change {
        # "Started one, Unique ID holds\nresponse"
        n260 = event-data() -> ()  [unwired: 1 in, 1 out]
        n261 = property on="Command Selection" class="MCListbox (strict)"() -> ("ItemNames"=w395:string[][])  [unwired: 2 in, 2 out]
        n262 = Index Array(array=w395, index (row)="Command Selection", index (col)=0) -> (element=w393:string)
        n263 = call <vilib>:"Invoke Commands.vi"("Command Params"="Command Params", "Function Name"=w393) -> ("Params"=w389:u8, "Started"=w388:bool)  [unwired: 7 in, 1 out]
        n264 = Array Subset(array="Command Params", length (row)=w389) -> (w390:string[][])  [unwired: 3 in]
        n265 = Select(t="Executing" ("Cmd Status"), s=w388, f="" ("Cmd Status")) -> (s? t:f=→"Cmd Status":string)
      }
      event "Command Selection": Double Click {
        n266 = event-data() -> ("Row"=w403:i32)  [unwired: 1 in]
        n267 = property on="Command Selection" class="MCListbox (strict)"() -> ("ItemNames"=w406:string[][])  [unwired: 2 in, 2 out]
        n268 = local read "Command Params"() -> (w402:string[][])
        n269 = Index Array(array=w406, index (row)=w403, index (col)=0) -> (element=w404:string)
        n270 = call <vilib>:"Invoke Commands.vi"("Command Params"=w402, "Function Name"=w404) -> ("Params"=w401:u8, "Started"=w396:bool)  [unwired: 7 in, 1 out]
        n271 = Array Subset(array=w402, length (row)=w401) -> (w400:string[][])  [unwired: 3 in]
        n272 = Select(t="Executing" ("Cmd Status"), s=w396, f="" ("Cmd Status")) -> (s? t:f=w397:string)
        n273 = local write "Cmd Status"(w397) -> ()
      }
      event "CheckList": Double Click {
        # "Shift clears all"
        # "Update symbols on the listbox"
        n274 = event-data() -> ("PlatMods.Shift"=w408:bool, "Row"=w410:i32)  [unwired: 1 in]
        n275 = case shown="True" w408 {
          tunnel: w410 -> [w414 _]
          tunnel: 1 -> [w413 _]
          frame False {
            n276 = property on="CheckList" class="LstBox (strict)"() -> ("Item Symbols"=w412:i32[])  [unwired: 2 in, 2 out]
            n277 = Replace Array Subset(array=w412, new element=w413, index=w414) -> (w411:i32[])
            n278 = property on="CheckList" class="LstBox (strict)"("Item Symbols"=w411) -> ()  [unwired: 2 in, 2 out]
          }
          frame True {
            w415 = 0 ("Top Row")
            n279 = property on="CheckList" class="LstBox (strict)"() -> ("Number of Rows"=w417:u32)  [unwired: 2 in, 2 out]
            n280 = Initialize Array(0, w417) -> (w416:i32[])
            n281 = property on="CheckList" class="LstBox (strict)"("Top Row"=w415, "Value"=w415, "Item Symbols"=w416) -> ()  [unwired: 2 in, 2 out]
          }
        }
      }
      event "CheckList": Key Down {
        # "Update symbols on the listbox\nLeft and right keys check and uncheck"
        n282 = event-data() -> ("VKey"=w421:T22)  [unwired: 1 in]
        n283 = case shown="\"Left\", \"Right\"" w421 {
          selector: w421 -> [w426 _]
          tunnel: eventvkey."Left" ("VKey") -> [w424 _]
          frame "Left", "Right" {
            n284 = Equal?(x=w424, y=w426) -> (x = y?=w425:bool)
            n285 = Select(t=0, s=w425, f=1) -> (s? t:f=w427:i32)
            n286 = property on="CheckList" class="LstBox (strict)"() -> ("Item Symbols"=w430:i32[])  [unwired: 2 in, 2 out]
            n287 = Replace Array Subset(array=w430, new element=w427, index="CheckList") -> (w429:i32[])
            n288 = property on="CheckList" class="LstBox (strict)"("Item Symbols"=w429) -> ()  [unwired: 2 in, 2 out]
          }
          frame Default {
          }
        }
      }
      event "Motor.Enable": Value Change {
        # "When the test mode otor enable helper is set, update that\ntree row item's value"
        n289 = event-data() -> ("NewVal"=w436:bool)  [unwired: 1 in]
        n290 = Unbundle("Motor") -> ("Value"=w435:dbl)  [unwired: 1 out]
        n291 = Select(t=w435, s=w436, f=0.0) -> (s? t:f=w433:dbl)
        n292 = call <vilib>:"NT Write Number.vi"("Numeric"=w433, "Name"=w432) -> ()  [unwired: 9 in, 1 out]
      }
      event "Test Slider": Value Change {
        # "When the test mode slider helper is set, update that\ntree row item's value"
        n293 = event-data() -> ("NewVal"=w439:dbl)  [unwired: 1 in]
        n294 = call <vilib>:"NT Write Number.vi"("Numeric"=w439, "Name"=w440) -> ()  [unwired: 9 in, 1 out]
      }
      event "On/Off": Value Change {
        # "When the test mode on/off helper value is set, update that\ntree row item's value"
        n295 = event-data() -> ("NewVal"=w444:bool)  [unwired: 1 in]
        n296 = Boolean To (0,1)(Boolean=w444) -> (0, 1=w443:i16)
        n297 = call <vilib>:"NT Write Number.vi"("Numeric"=w443, "Name"=w442) -> ()  [unwired: 9 in, 1 out]
      }
      event "Rev/Fwd": Value Change {
        # "When the test mode helper value for relays is set, update that\ntree row item's value"
        n298 = event-data() -> ("NewVal.Forward"=w452:bool, "NewVal.Reverse"=w451:bool)  [unwired: 1 in]
        n299 = Boolean To (0,1)(Boolean=w452) -> (0, 1=w448:i16)
        n300 = Boolean To (0,1)(Boolean=w451) -> (0, 1=w450:i16)
        n301 = Negate(x=w450) -> (-x=w449:i16)
        n302 = Add(x=w448, y=w449) -> (x+y=w447:i16)
        n303 = call <vilib>:"NT Write Number.vi"("Numeric"=w447, "Name"=w446) -> ()  [unwired: 9 in, 1 out]
      }
      event "Test Ring": Value Change {
        # "When a test mode helper value is selected from the ring,\nset the tree item's variable to the string value"
        n304 = event-data() -> ("NewVal"=w456:u16)  [unwired: 1 in]
        n305 = property on="Test Ring" class="Ring (strict)"() -> ("Strings []"=w457:string[])  [unwired: 2 in, 2 out]
        n306 = Index Array(array=w457, index=w456) -> (element=w455:string)
        n307 = call <vilib>:"NT Write String.vi"("String"=w455, "Name"=w454) -> ()  [unwired: 9 in, 1 out]
      }
      event "Rec Mode": Value Change {
        # "Update globals for recording mode and path to read log from.\nClear when logging and let NetworkTables set path for vision to\nuse."
        n308 = event-data() -> ("NewVal"=w468:enum32{"Stop", "Record", "Playback"})  [unwired: 1 in]
        n309 = global write "WPI_DashboardLogging Global.vi" "Logging Filename"(path "") -> ()
        n310 = global write "WPI_DashboardLogging Global.vi" "Recording"(w468) -> ()
        n311 = case shown="\"Playback\"" w468 {
          tunnel: w467 -> [_ w470 w479]
          tunnel: [_ _ w478] -> w465
          tunnel: [_ _ w477] -> _
          tunnel: w463 -> [_ _ w475]
          tunnel: cluster{i32, i32} {-250, 170} -> [_ _ w474]
          tunnel: [_ _ T23 {"Image Size"=TRUE, "Image Type"=TRUE, "Pixel Value"=TRUE, "ROI Information"=TRUE, "Zoom Factor"=FALSE} ("Image Information Shown:All Elements")] -> w458
          tunnel: [_ _ TRUE ("Zoom Factor")] -> w459
          tunnel: w461 -> [_ _ w471]
          frame Default {
          }
          frame "Stop", "Record" {
            # "Place Window too"
            n312 = invoke class="VI" method="FP.Close"(reference=w470) -> (reference out=w469:refnum<vi>)  [unwired: 2 in, 2 out]
            n313 = invoke class="VI" method="Abort VI"(reference=w469) -> ()  [unwired: 2 in, 3 out]
          }
          frame "Playback" {
            n314 = call "Open Playback Panel.vi"("Offset"=w474, "DB VI Ref"=w475, "Playback in"=w479) -> ("Playback out"=w476:refnum<vi>)  [unwired: 8 in]
            n315 = register-events(w476, w471) -> (reference out=w478:refnum<event-registration>, error out=w477:errorcluster)  [unwired: 2 in]
          }
        }
        n316 = property on="Camera Image" class="ImageControl"("Image Information Shown"=w458, "Image Information Visible"=w459) -> ()  [unwired: 2 in, 2 out]
        n317 = property on="Camera Image Right" class="ImageControl"("Image Information Shown"=w458, "Image Information Visible"=w459) -> ()  [unwired: 2 in, 2 out]
        n318 = call <vilib>:"WPI_DashboardNT Log FieldName Cache.vi"("Operation"=enum16{"Lookup/Add", "Index", "Clear"}."Clear") -> ()  [unwired: 8 in, 3 out]
      }
      event Panel Close {
        w481 = enum32{"Stop", "Record", "Playback"}."Stop" ("Rec Mode")
        # "Playback window has been closed, abort"
        n319 = event-data() -> ()  [unwired: 1 in, 4 out]
        n320 = local write "Rec Mode"(w481) -> ()
        n321 = global write "WPI_DashboardLogging Global.vi" "Recording"(w481) -> ()
      }
      event Panel Close {
        # "Abort playback window and ourself"
        n322 = event-data() -> ()  [unwired: 1 in, 4 out]
        n323 = invoke class="VI" method="FP.Close"(reference=w485) -> (reference out=w484:refnum<vi>)  [unwired: 2 in, 2 out]
        n324 = invoke class="VI" method="Abort VI"(reference=w484) -> (error out=w483:errorcluster)  [unwired: 2 in, 2 out]
        n325 = invoke class="VI" method="Abort VI"(error in=w483) -> ()  [unwired: 2 in, 3 out]
      }
      event User Event {
        n326 = event-data() -> ("IDs"=w492:cluster{"RPC field ID":u16, "Unique ID":u16}, "String"=w491:string)  [unwired: 1 in]
        n327 = local write "Cmd Status"("" ("Cmd Status")) -> ()
        n328 = Bundle("IDs"=w492, "String"=w491) -> (w490:T9)  [unwired: 1 in]
        n329 = call <vilib>:"Retrieve RPC Response.vi"("RPC Response"=w490) -> ("Output"=w488:string[][])  [unwired: 10 in]
        n330 = Build Array (concatenate)(w486, w488) -> (w487:string[][])
        n331 = local write "Command Params"(w487) -> ()
      }
      event "Tree": Double Click {
        n332 = event-data() -> ("PlatMods"=w498:T26, "Tag"=w495:string)  [unwired: 1 in]
        n333 = Unbundle(w498) -> ("Shift"=w497:bool)  [unwired: 4 out]
        n334 = Not(x=w497) -> (.not. x?=w496:bool)
        n335 = String Subset(string=w495, length (rest)=1 ("length (rest)")) -> (substring=w494:string)  [unwired: 1 in]
        n336 = case shown="\"/\"" w494 {
          tunnel: w495 -> [_ w501]
          tunnel: w496 -> [_ w500]
          frame Default {
          }
          frame "/" {
            n337 = call <vilib>:"NT Update Persistence.vi"("Persistence"=w500, "Name"=w501) -> ()  [unwired: 9 in, 1 out]
          }
        }
      }
    }
  }
  n338 = while {
    tunnel: w55 -> [w513]
    tunnel: w36 -> [w511]
    tunnel: [w509] -> _
    tunnel: u32 1000 ("milliseconds to wait") -> [w508]
    tunnel: w26 -> [w502]
    i -> [w509]
    stop <- FALSE stop-if-true
    n339 = Wait on Notification(notifier=w511, timeout in ms (-1)=w508) -> (notification=w510:string, timed out?=w506:bool)  [unwired: 2 in, 2 out]
    n340 = local read "Rec Mode"() -> (w504:enum32{"Stop", "Record", "Playback"})
    n341 = Equal?(x=w504, y=u16 2 ("Rec Mode")) -> (x = y?=w505:bool)
    n342 = Compound Arithmetic op=OR(invert w506, w505) -> (w507:bool)
    n343 = case shown="True" w507 {
      tunnel: w513 -> [_ w516]
      tunnel: w510 -> [_ w515]
      tunnel: w502 -> [_ w514]
      frame False {
      }
      frame True {
        n344 = call <vilib>:"Bind Controls to SmartDashboard.vi"("RPC ref"=w514, "Bound Control Refs"=w516, "Server IP Address"=w515) -> ()  [unwired: 9 in]
      }
    }
  }
